vi "marshalling.vi"(8 "error in (no error)":errorcluster, 10 "Variant":variant, 11 "Serializer":refnum<class "Serializer.JSON.lvclass">) -> (0 "error out":errorcluster, 2 "JSON String":string, 3 "Serializer out":refnum<class "Serializer.JSON.lvclass">)   [LabVIEW 2013, in "OpenSerializer.JKI-JSON.lvlib" / "Serializer.JSON.lvclass"]
uses:
  Serializer.JSON.lvclass
  Serializer.JSON.lvclass/Serializer.JSON.ctl
  <vilib>/addons/_JKI.lib/Serialization/JSON/JKI JSON Serialization.lvlib
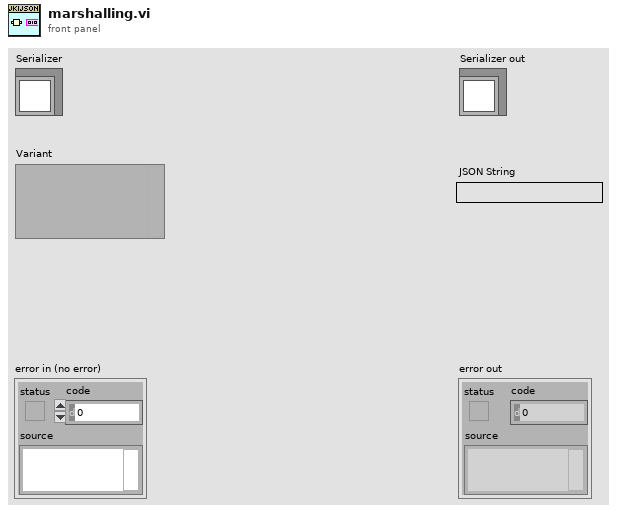
[diagram p1: front panel]
types:
  T1 = typedef "JKI JSON Serialization.lvlib/Timestamp Options.ctl" = cluster{"Convert Timestamps":bool, "UTC":bool}
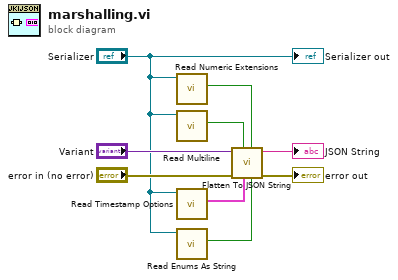
[diagram p0: block diagram]
diagram:
  n1 = call "Read Numeric Extensions.vi"("Serializer.JSON in"="Serializer") -> ("Numeric Extensions"=w1:bool)  [unwired: 9 in, 1 out]
  n2 = call "Read Multiline.vi"("Serializer.JSON in"="Serializer") -> ("Multiline"=w3:bool)  [unwired: 9 in, 1 out]
  n3 = call "Read Timestamp Options.vi"("Serializer.JSON in"="Serializer") -> ("Timestamp Serialization"=w5:T1)  [unwired: 9 in, 1 out]
  n4 = call "Read Enums As String.vi"("Serializer.JSON in"="Serializer") -> ("Enums As String"=w4:bool)  [unwired: 9 in, 1 out]
  n5 = call <vilib>:"Flatten To JSON String.vi"("Enums As String (F)"=w4, "Numeric Extensions (F)"=w1, "Timestamp Options"=w5, "Multiline (T)"=w3, "error in (no error)"="error in (no error)", "Variant"="Variant") -> ("error out"=→"error out":errorcluster, "JSON String"=→"JSON String":string)  [unwired: 4 in]
  "Serializer out" <- "Serializer"
